vi "GetNextInterval.vi"(8 "error in":errorcluster, 11 "VISA resource name":refnum<visa-resource-name>) -> (0 "error out":errorcluster, 1 "Next interval":i32, 2 "Next interval string":string, 3 "VISA resource name out":refnum<visa-resource-name>)   [LabVIEW 2023, in "Thermotron 8800.lvlib"]
doc: "NXTI\nCommand name: Send next interval\nCommand type: Program status\nDescription: Queries the 8800 for the next interval that will be executed. The 8800 sends an integer indicating the next interval number.\nSyntax: NXTI?\nData type: Integer\nQuery example: NXTI?\n8800 response: 5 (The next interval that will be executed is interval 5.)"
uses:
  Thermotron 8800.lvlib
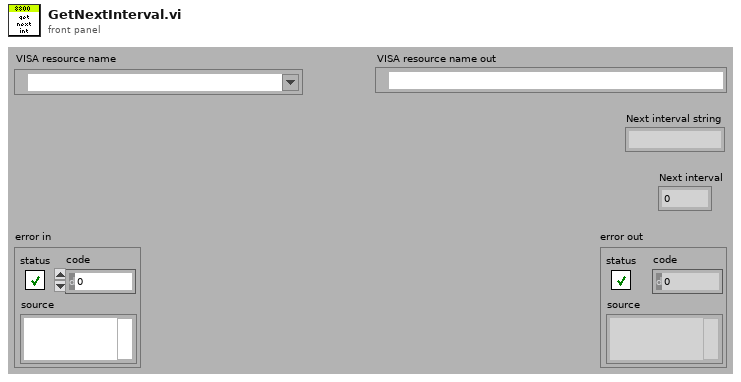
[diagram p1: front panel]
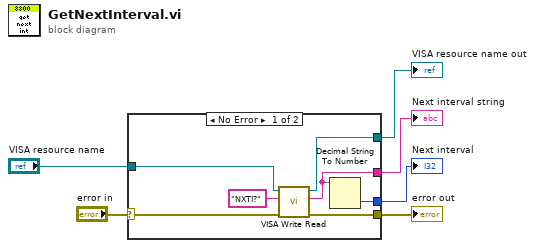
[diagram p0: block diagram]
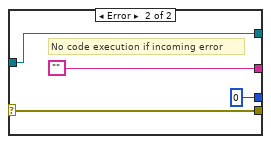
[diagram p2: hidden frame]
diagram:
  n1 = case shown="No Error" "error in" {
    selector: "error in" -> [w13 w17]
    tunnel: [w12 w17] -> w5
    tunnel: "VISA resource name" -> [w11 w14]
    tunnel: [w10 w14] -> w3
    tunnel: [w9 ""] -> w1
    tunnel: [w8 0] -> w2
    frame No Error {
      n2 = call "VISA Write Read.vi"("error in (no error)"=w13, "8800 Command"="NXTI?", "VISA Refnum in"=w11) -> ("error out"=w12:errorcluster, "read buffer"=w9:string, "VISA Refnum out"=w10:refnum<visa-resource-name>)  [unwired: 6 in]
      n3 = Decimal String To Number(string=w9) -> (number=w8:i32)  [unwired: 2 in, 1 out]
    }
    frame Error {
      # "No code execution if incoming error"
    }
  }
  "error out" <- w5
  "VISA resource name out" <- w3
  "Next interval" <- w2
  "Next interval string" <- w1
